vi "fgv_Chirp Paremeters Sweep.vi"(8 "error in":errorcluster, 9 "Function":T1, 11 "Z-stack Chirp parameters (all Z planes) in":cluster{"HexPackets":string[]}[](array[cluster])) -> (0 "error out":errorcluster, 3 "Z-stack Chirp parameters (all Z planes)":cluster{"HexPackets":string[]}[](array[cluster]))   [LabVIEW 2017]
uses:
  Typedefs/Read Write Enum.ctl
panel:
  # "SUBROUTINE"
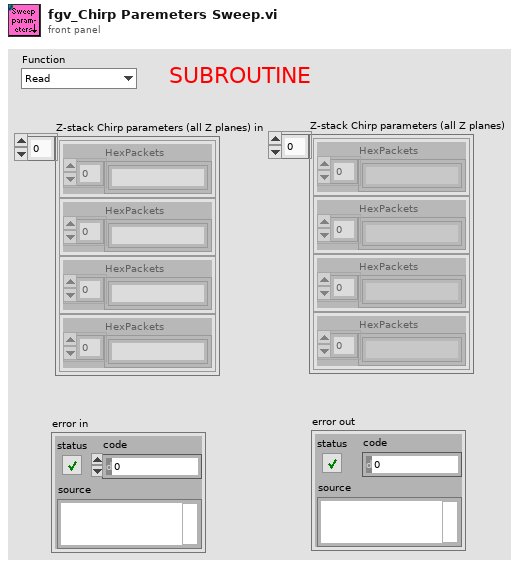
[diagram p1: front panel]
types:
  T1 = typedef "Read Write Enum.ctl" = enum16{"Read", "Write"}
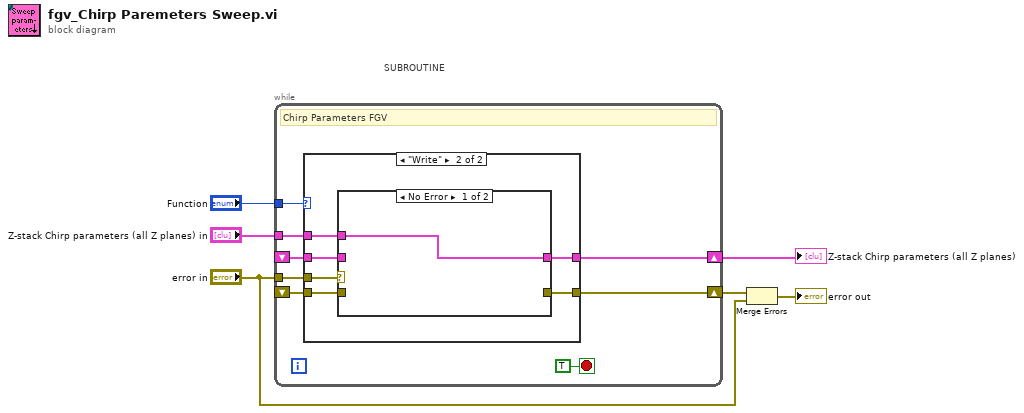
[diagram p0: block diagram]
diagram:
  # "SUBROUTINE"
  n1 = while {
    tunnel: "Function" -> [w13]
    tunnel: "Z-stack Chirp parameters (all Z planes) in" -> [w12]
    shift-right: [w11] -> w4
    shift-left: _ -> [w10]
    tunnel: "error in" -> [w9]
    shift-right: [w8] -> w3
    shift-left: _ -> [w7]
    stop <- TRUE stop-if-true
    # "Chirp Parameters FGV"
    n2 = case shown="\"Write\"" w13 {
      tunnel: w12 -> [_ w21]
      tunnel: [w16 w20] -> w11
      tunnel: w10 -> [w16 w19]
      tunnel: w9 -> [_ w22]
      tunnel: [w15 w18] -> w8
      tunnel: w7 -> [w15 w17]
      frame "Read", Default {
      }
      frame "Write" {
        n3 = case shown="No Error" w22 {
          selector: w22 -> [_ w24]
          tunnel: w21 -> [w23 _]
          tunnel: [w23 w25] -> w20
          tunnel: w19 -> [_ w25]
          tunnel: [_ w24] -> w18
          tunnel: w17 -> [_ _]
          frame No Error {
          }
          frame Error {
          }
        }
      }
    }
  }
  "Z-stack Chirp parameters (all Z planes)" <- w4
  n4 = Merge Errors(w3, "error in") -> (→"error out":errorcluster)
